vi "svx_SC Line Image.vi"(4 "Boundary Color":u32(colorbox), 5 "shaft rotating direction":u16(ring) items=["CCW", "CW"], 6 "Arrow Color":u32(colorbox)=10184, 7 "SC Line in":refnum<vi>, 9 "start point":enum16{"center", "top", "bottom"}(ring), 10 "boundary":cluster{"x axis":dbl, "y axis":dbl}, 11 "Picture in":picture) -> ()   [LabVIEW 2017, in "SVX SC Line.xctl"]
uses:
  <vilib>/addons/_XControls/Shaft Centerline/SVX SC Line.xctl
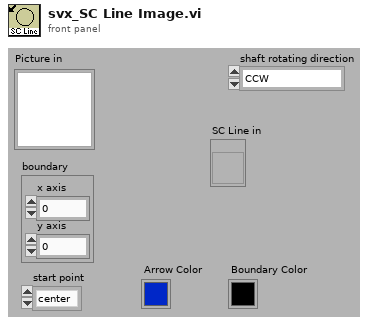
[diagram p1: front panel]
types:
  T1 = typedef "LVBoundsTypeDef.ctl" = cluster{"Width":u32, "Height":u32}
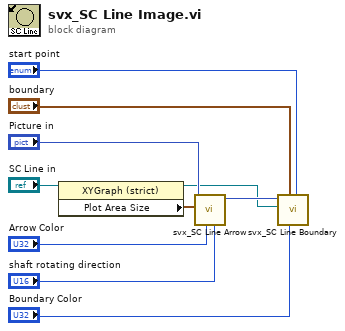
[diagram p0: block diagram]
diagram:
  n1 = property class="XYGraph (strict)"(reference="SC Line in") -> (reference out=w5:refnum<vi>, "Plot Area Size"=w8:T1)  [unwired: 1 in, 1 out]
  n2 = call <vilib>:"svx_SC Line Arrow.vi"("shaft rotating direction"="shaft rotating direction", "color"="Arrow Color", "Plot Area:Size"=w8, "Picture in"="Picture in") -> ("new picture"=w6:picture)  [unwired: 6 in, 1 out]
  n3 = call <vilib>:"svx_SC Line Boundary.vi"("start point"="start point", "Boundary Color"="Boundary Color", "boundary"="boundary", "Shaft Centerline"=w5, "Picture in"=w6) -> ()  [unwired: 6 in, 1 out]
